vi "Get Motors Position.vi"(8 "error in (no error)":errorcluster, 11 "KUKA youBot gripper in":refnum<class "NI_Robotics_KUKA youBot Gripper.lvclass">) -> (0 "error out":errorcluster, 2 "position (m)":dbl[](array[numeric]), 3 "KUKA youBot gripper out":refnum<class "NI_Robotics_KUKA youBot Gripper.lvclass">)   [LabVIEW 2017, in "NI_Robotics_KUKA youBot Host.lvlib" / "NI_Robotics_KUKA youBot Gripper.lvclass"]
doc: "Gets the motors position, which the position encoder senses, of the joints of a KUKA youBot gripper."
uses:
  <vilib>/robotics/KUKA youBot/Basic Device/Gripper/NI_Robotics_KUKA youBot Gripper.lvclass
  <vilib>/robotics/KUKA youBot/Basic Device/Gripper/NI_Robotics_KUKA youBot Gripper.lvclass/NI_Robotics_KUKA youBot Gripper.ctl
  <vilib>/robotics/KUKA youBot/Motor/Gripper Motor/NI_Robotics_KUKA youBot Gripper Motor.lvclass
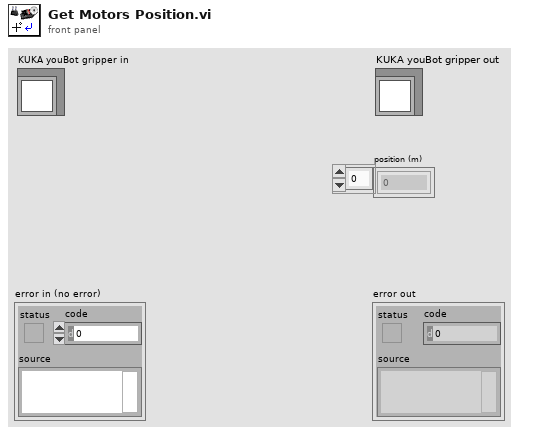
[diagram p1: front panel]
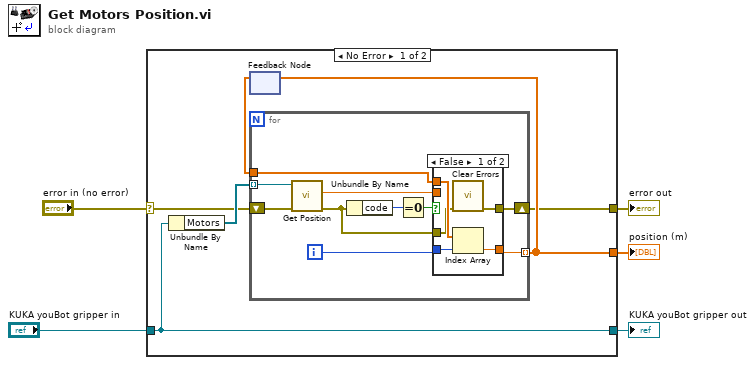
[diagram p0: block diagram]
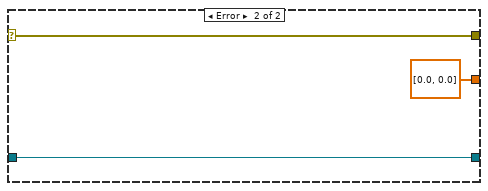
[diagram p3: hidden frame]
diagram:
  n1 = case shown="No Error" "error in (no error)" {
    selector: "error in (no error)" -> [w9 w31]
    tunnel: [w6 w31] -> w4
    tunnel: [w11 w30] -> w2
    tunnel: "KUKA youBot gripper in" -> [w11 w30]
    tunnel: [w8 dbl[] [0.0, 0.0]] -> w1
    frame No Error {
      n2 = Unbundle By Name(w11) -> ("Motors"=w10:refnum<class "NI_Robotics_KUKA youBot Gripper Motor.lvclass">[])
      n3 = feedback #1() -> (w7:dbl[])  [unwired: 1 in]
      n4 = for {
        tunnel: w10 -> [w21] mode=indexing
        shift-right: [w16] -> w6
        shift-left: w9 -> [w20]
        tunnel: [w18] -> w8 mode=indexing
        tunnel: w7 -> [w19]
        i -> [w15]
        n5 = call-dynamic "Get Position.vi"("error in (no error)"=w20, "KUKA youBot gripper motor in"=w21) -> ("error out"=w12:errorcluster, "position (m)"=w17:dbl)  [unwired: 7 in, 1 out]
        n6 = Unbundle By Name(w12) -> ("code"=w13:i32)
        n7 = Equal To 0?(x=w13) -> (x = 0?=w14:bool)
        n8 = case shown="False" w14 {
          tunnel: w19 -> [w25 _]
          tunnel: [w23 w28] -> w18
          tunnel: w17 -> [_ w28]
          tunnel: [w26 w27] -> w16
          tunnel: w15 -> [w24 _]
          tunnel: w12 -> [w22 w27]
          frame False {
            n9 = call <vilib>:"Clear Errors.vi"("error in (no error)"=w22) -> ("error out"=w26:errorcluster)  [unwired: 5 in, 1 out]
            n10 = Index Array(array=w25, index=w24) -> (element=w23:dbl)
          }
          frame True {
          }
        }
      }
      n11 = feedback-in #1(w8) -> ()
    }
    frame Error {
    }
  }
  "error out" <- w4
  "KUKA youBot gripper out" <- w2
  "position (m)" <- w1
